vi "subVI_Strain_Peak.vi"(8 "error in (no error)":errorcluster caption="에러 입력(에러 없음)", 11 "Data_in":dbl[][](array[numeric])) -> (0 "error out":errorcluster caption="에러 출력", 2 "Peak Strain":dbl, 3 "Data_out":dbl[][](array[numeric]))   [LabVIEW 2013]
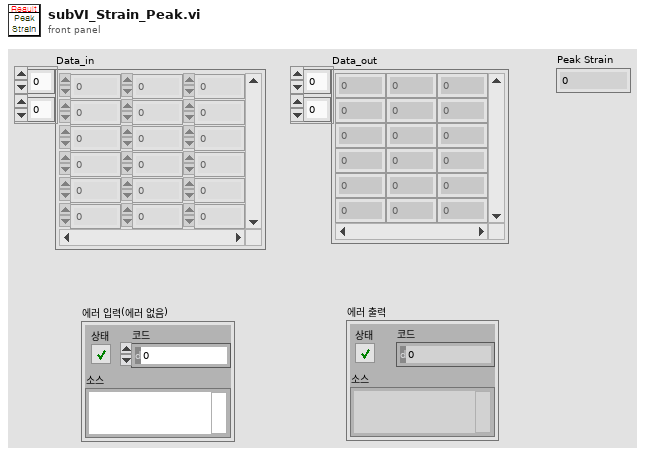
[diagram p1: front panel]
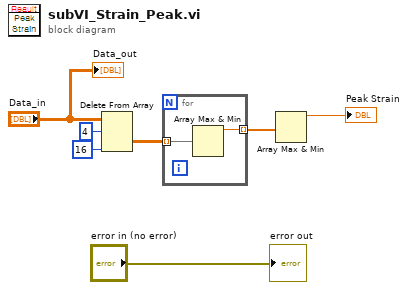
[diagram p0: block diagram]
diagram:
  n1 = Delete From Array(array="Data_in", length=4 ("길이"), index (row)=16 ("인덱스 (행)")) -> (deleted portion=w5:dbl[][])  [unwired: 1 in, 1 out]
  n2 = for {
    tunnel: w5 -> [w9] mode=indexing
    tunnel: [w8] -> w4 mode=indexing
    n3 = Array Max & Min(array=w9) -> (max value=w8:dbl)  [unwired: 3 out]
  }
  n4 = Array Max & Min(array=w4) -> (max value=→"Peak Strain":dbl)  [unwired: 3 out]
  "Data_out" <- "Data_in"
  "error out" <- "error in (no error)"
